vi "getEEPROMvector.vi"(10 "vectorName":string, 11 "EEPROM_Settings":string) -> (0 "error out":errorcluster, 3 "vectorOut":cluster{dbl, dbl, dbl})   [LabVIEW 2015]
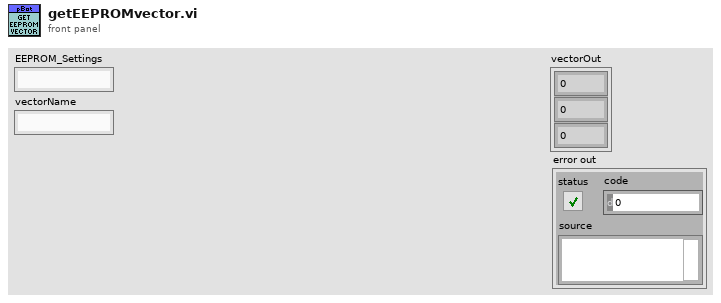
[diagram p1: front panel]
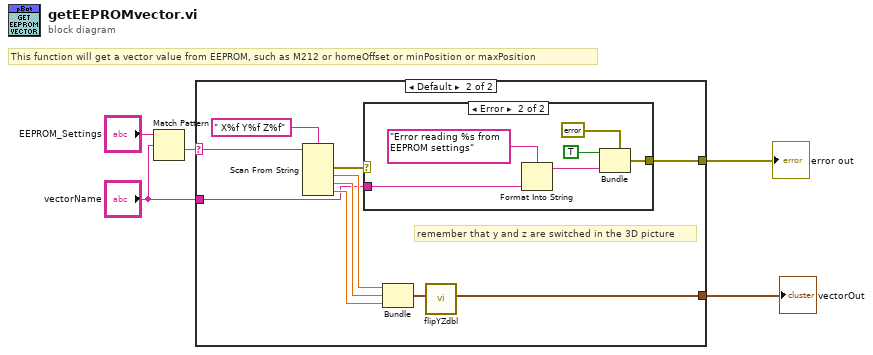
[diagram p0: block diagram]
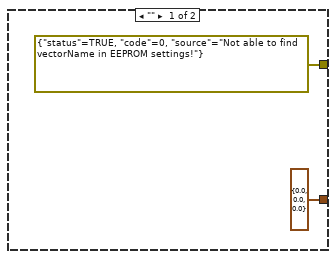
[diagram p2: hidden frame]
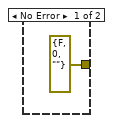
[diagram p3: hidden frame]
diagram:
  # "This function will get a vector value from EEPROM, such as M212 or homeOffset or minPosition or maxPosition"
  n1 = Match Pattern(string="EEPROM_Settings", regular expression="vectorName") -> (after substring=w4:string)  [unwired: 1 in, 3 out]
  n2 = case shown="Default" w4 {
    selector: w4 -> [_ w16]
    tunnel: [cluster{dbl, dbl, dbl} {0.0, 0.0, 0.0} w11] -> w3
    tunnel: [errorcluster {"status"=TRUE, "code"=0, "source"="Not able to find vectorName in EEPROM settings!"} ("error constant") w9] -> w2
    tunnel: "vectorName" -> [_ w8]
    frame "" {
    }
    frame Default {
      # "remember that y and z are switched in the 3D picture"
      n3 = Scan From String(format string=" X%f Y%f Z%f", input string=w16) -> (error out=w10:errorcluster, output 1=w15:dbl, output 2=w14:dbl, output 3=w13:dbl)  [unwired: 5 in, 2 out]
      n4 = case shown="Error" w10 {
        tunnel: [errorcluster {"status"=FALSE, "code"=0, "source"=""} ("error constant") w19] -> w9
        tunnel: w8 -> [_ w23]
        frame No Error {
        }
        frame Error {
          n5 = Format Into String(format string="Error reading %s from EEPROM settings", w23) -> (resulting string=w21:string)  [unwired: 2 in, 1 out]
          n6 = Bundle(cluster=errorcluster {"status"=TRUE, "code"=0, "source"=""} ("error constant"), "status"=TRUE, "source"=w21) -> (w19:errorcluster)  [unwired: 1 in]
        }
      }
      n7 = Bundle(w15, w14, w13) -> (w12:cluster{dbl, dbl, dbl})  [unwired: 1 in]
      n8 = call "flipYZdbl.vi"("pointIn"=w12) -> ("pointOut"=w11:cluster{"X":dbl, "Y":dbl, "Z":dbl})  [unwired: 10 in]
    }
  }
  "error out" <- w2
  "vectorOut" <- w3
